vi "Read Registration Complete.vi"(8 "error in (no error)":errorcluster, 11 "File Actor in":refnum<class "File Actor.lvclass">) -> (0 "error out":errorcluster, 2 "Registration Complete":bool, 3 "File Actor out":refnum<class "File Actor.lvclass">)   [LabVIEW 2017, in "File Library.lvlib" / "File Actor.lvclass"]
uses:
  File Actor.lvclass
  File Actor.lvclass/File Actor.ctl
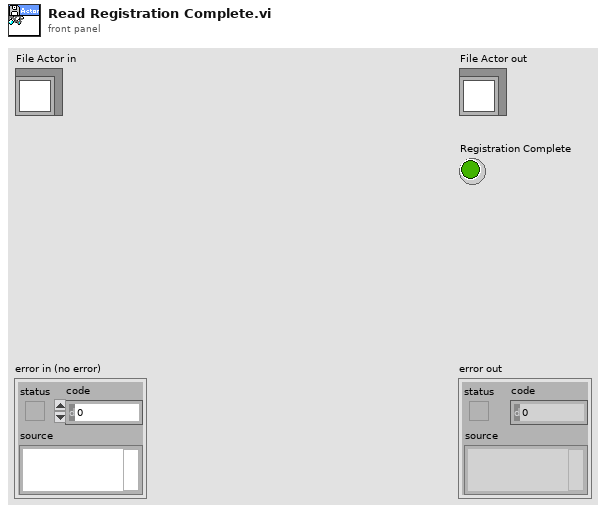
[diagram p1: front panel]
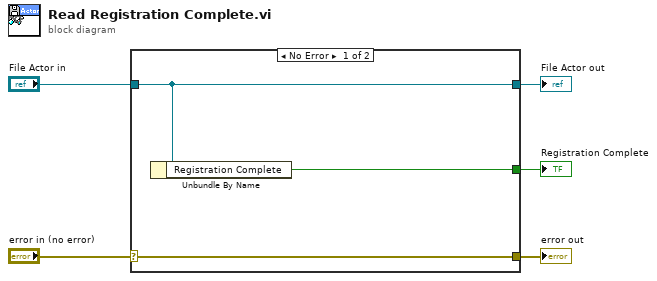
[diagram p0: block diagram]
diagram:
  n1 = case shown="No Error" "error in (no error)" {
    selector: "error in (no error)" -> [w8 w9]
    tunnel: [w8 w9] -> w4
    tunnel: [w7 w10] -> w2
    tunnel: "File Actor in" -> [w7 w10]
    tunnel: [w6 _] -> w1
    frame No Error {
      n2 = Unbundle By Name(w7) -> ("Registration Complete"=w6:bool)
    }
    frame Error {
    }
  }
  "error out" <- w4
  "File Actor out" <- w2
  "Registration Complete" <- w1
